vi "oa_Build Data from Order Magnitude and Phase.vi"(5 "reset? (F)":bool, 6 "samples/revolution wanted":dbl=4.0 format="%.2f", 7 "order":dbl=1.0 format="%.2f", 8 "error in (no error)":errorcluster, 9 "samples/revolution":dbl=1.0 format="%.2f", 10 "phase lag":dbl[][](array[numeric]) format="%.2f", 11 "magnitude":dbl[][](array[numeric]) format="%.2f") -> (0 "error out":errorcluster, 2 "actual samples/rev":dbl=1.0 format="%.2f", 3 "order waveform":dbl[][](array[numeric]) format="%.2f")   [LabVIEW 2017]
uses:
  <vilib>/addons/Sound and Vibration/Order Analysis/Resample Order Tracking/SoundVib_Resampling.lvlib
  <vilib>/Analysis/NI_AALPro.lvlib
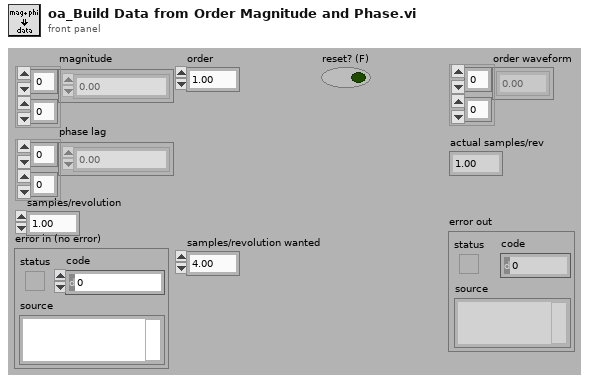
[diagram p1: front panel]
types:
  T1 = typedef "OAT Decimation Filter.ctl" = cluster{"coefficients":dbl[], "factor":i32}
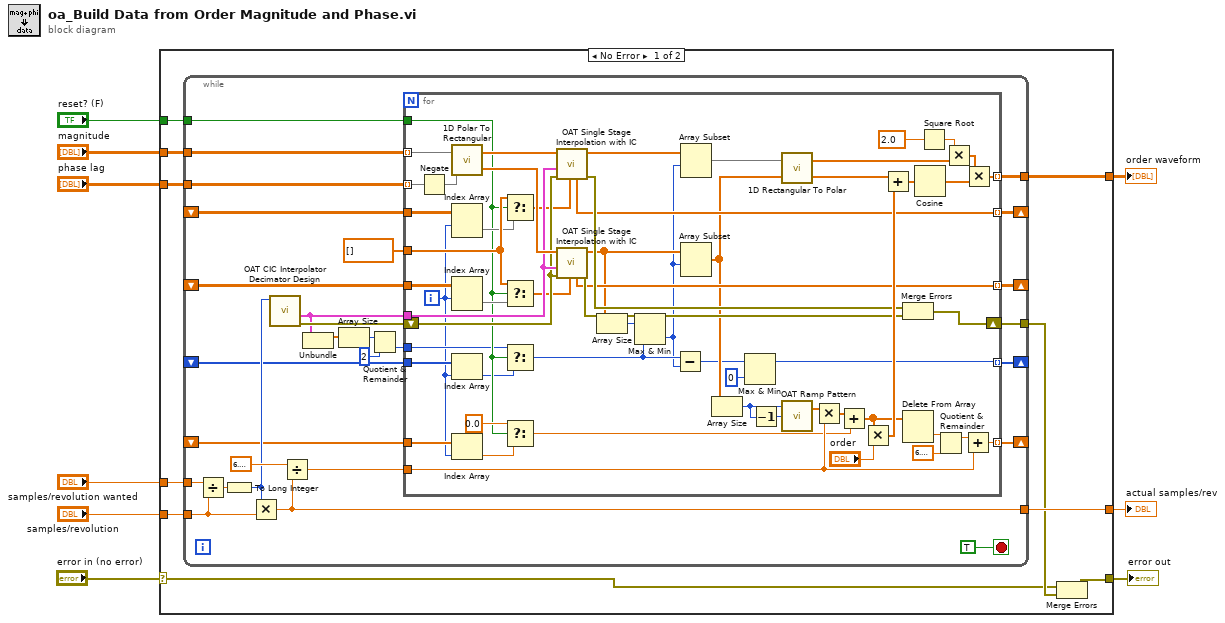
[diagram p0: block diagram]
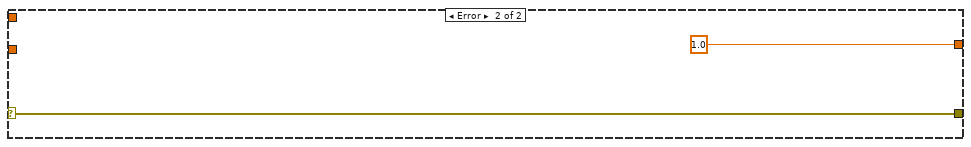
[diagram p2: hidden frame]
diagram:
  n1 = case shown="No Error" "error in (no error)" {
    selector: "error in (no error)" -> [w10 w107]
    tunnel: "samples/revolution wanted" -> [w19 _]
    tunnel: "samples/revolution" -> [w18 _]
    tunnel: [w17 _] -> w7
    tunnel: "magnitude" -> [w16 _]
    tunnel: [w11 w107] -> w5
    tunnel: [w15 1.0] -> w4
    tunnel: "phase lag" -> [w14 _]
    tunnel: "reset? (F)" -> [w13 _]
    frame No Error {
      n2 = while {
        tunnel: w19 -> [w47]
        tunnel: w18 -> [w45]
        tunnel: [w42] -> w17
        tunnel: w16 -> [w41]
        tunnel: [w39] -> w12
        tunnel: [w38] -> w15
        tunnel: w14 -> [w37]
        shift-right: [w34] -> _
        shift-left: _ -> [w33]
        tunnel: w13 -> [w32]
        shift-right: [w30] -> _
        shift-left: _ -> [w29]
        shift-right: [w28] -> _
        shift-left: _ -> [w27]
        shift-right: [w21] -> _
        shift-left: _ -> [w20]
        stop <- TRUE stop-if-true
        n3 = Divide(x=w47, y=w45) -> (x/y=w46:dbl)
        n4 = To Long Integer(number=w46) -> (32bit integer=w43:i32)
        n5 = Multiply(x=w43, y=w45) -> (x*y=w38:dbl)
        n6 = call <vilib>:"OAT CIC Interpolator Decimator Design.vi"("interpolation/decimation factor"=w43) -> ("error out"=w40:errorcluster, "filter"=w23:T1)  [unwired: 9 in]
        n7 = Divide(x=6.283185307179586, y=w38) -> (x/y=w35:dbl)
        n8 = Unbundle(w23) -> ("coefficients"=w26:dbl[])  [unwired: 1 out]
        n9 = Array Size(array=w26) -> (size(s)=w25:i32)
        n10 = Quotient & Remainder(x=w25, y=2) -> (floor(x/y)=w22:i32)  [unwired: 1 out]
        n11 = for {
          tunnel: w23 -> [w77]
          tunnel: [w96] -> w42 mode=indexing
          tunnel: w41 -> [w95] mode=indexing
          tunnel: w37 -> [w91] mode=indexing
          tunnel: w35 -> [w87]
          tunnel: [w86] -> w34 mode=indexing
          tunnel: w33 -> [w64]
          tunnel: w32 -> [w58]
          shift-right: [w93] -> w39
          shift-left: w40 -> [w76]
          tunnel: dbl[] [] ("initial state") -> [w70]
          tunnel: [w71] -> w30 mode=indexing
          tunnel: w29 -> [w69]
          tunnel: [w67] -> w28 mode=indexing
          tunnel: w27 -> [w66]
          tunnel: w22 -> [w57]
          tunnel: [w52] -> w21 mode=indexing
          tunnel: w20 -> [w51]
          i -> [w50]
          n12 = Negate(x=w91) -> (-x=w80:dbl[])
          n13 = call <vilib>:"1D Polar To Rectangular.vi"("Magnitude"=w95, "Phase"=w80) -> ("X"=w79:dbl[], "Y"=w78:dbl[])  [unwired: 1 out]
          n14 = Index Array(array=w69, index (row)=w50) -> (element=w68:dbl[])  [unwired: 1 in]
          n15 = Index Array(array=w66, index (row)=w50) -> (element=w65:dbl[])  [unwired: 1 in]
          n16 = Index Array(array=w51, index=w50) -> (element=w49:i32)
          n17 = Index Array(array=w64, index=w50) -> (element=w63:dbl)
          n18 = Select(t=w70, s=w58, f=w68) -> (s? t:f=w73:dbl[])
          n19 = Select(t=w70, s=w58, f=w65) -> (s? t:f=w72:dbl[])
          n20 = Select(t=w57, s=w58, f=w49) -> (s? t:f=w55:i32)
          n21 = Select(t=0.0, s=w58, f=w63) -> (s? t:f=w82:dbl)
          n22 = call <vilib>:"OAT Single Stage Interpolation with IC.vi"("initial state"=w73, "error in (no error)"=w76, "filter"=w77, "X"=w79) -> ("error out"=w74:errorcluster, "Y"=w62:dbl[], "final state"=w71:dbl[])  [unwired: 5 in]
          n23 = call <vilib>:"OAT Single Stage Interpolation with IC.vi"("initial state"=w72, "error in (no error)"=w76, "filter"=w77, "X"=w78) -> ("error out"=w75:errorcluster, "Y"=w59:dbl[], "final state"=w67:dbl[])  [unwired: 5 in]
          n24 = Array Size(array=w59) -> (size(s)=w56:i32)
          n25 = Max & Min(x=w56, y=w55) -> (min(x,y)=w48:i32)  [unwired: 1 out]
          n26 = Subtract(x=w55, y=w48) -> (x-y=w54:i32)
          n27 = Array Subset(array=w62, index=w48) -> (w61:dbl[])  [unwired: 1 in]
          n28 = Array Subset(array=w59, index=w48) -> (w60:dbl[])  [unwired: 1 in]
          n29 = Array Size(array=w60) -> (size(s)=w81:i32)
          n30 = Max & Min(x=w54, y=0) -> (max(x,y)=w52:i32)  [unwired: 1 out]
          n31 = Decrement(x=w81) -> (x-1=w105:i32)
          n32 = call <vilib>:"1D Rectangular To Polar.vi"("X"=w61, "Y"=w60) -> ("Magnitude"=w98:dbl[], "Phase"=w99:dbl[])  [unwired: 1 out]
          n33 = call <vilib>:"OAT Ramp Pattern.vi"("end"=w105, "samples"=w81) -> ("Ramp Pattern"=w97:dbl[])  [unwired: 1 in, 1 out]
          n34 = Multiply(x=w97, y=w87) -> (x*y=w85:dbl[])
          n35 = Add(x=w85, y=w82) -> (x+y=w84:dbl[])
          n36 = Multiply(x=w84, y="order") -> (x*y=w102:dbl[])
          n37 = Add(x=w99, y=w102) -> (x+y=w101:dbl[])
          n38 = Merge Errors(w74, w75) -> (w93:errorcluster)
          n39 = Delete From Array(array=w84) -> (deleted portion=w90:dbl)  [unwired: 2 in, 1 out]
          n40 = Cosine(x=w101) -> (cos(x)=w100:dbl[])
          n41 = Square Root(x=2.0) -> (sqrt(x)=w103:dbl)
          n42 = Quotient & Remainder(x=w90, y=6.283185307179586) -> (x-y*floor(x/y)=w88:dbl)  [unwired: 1 out]
          n43 = Multiply(x=w103, y=w98) -> (x*y=w92:dbl[])
          n44 = Add(x=w88, y=w87) -> (x+y=w86:dbl)
          n45 = Multiply(x=w92, y=w100) -> (x*y=w96:dbl[])
        }
      }
      n46 = Merge Errors(w10, w12) -> (w11:errorcluster)
    }
    frame Error {
    }
  }
  "order waveform" <- w7
  "actual samples/rev" <- w4
  "error out" <- w5
